vi "oa_FIR Preprocess Filter dB to Linear.vi"(1 "dB value":dbl) -> (0 "linear value":dbl)   [LabVIEW 2017, in "SoundVib_RefDataProcess.lvlib"]
uses:
  <vilib>/addons/Sound and Vibration/Order Analysis/Referece Data Processing/SoundVib_RefDataProcess.lvlib
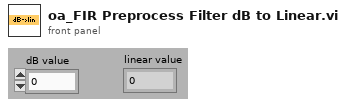
[diagram p1: front panel]
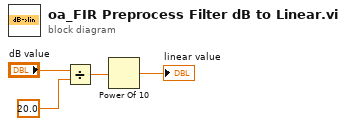
[diagram p0: block diagram]
diagram:
  n1 = Divide(x="dB value", y=20.0) -> (x/y=w2:dbl)
  n2 = Power Of 10(x=w2) -> (10^x=→"linear value":dbl)
